vi "ExecutePlay.vi"(0 "object in":refnum<class "StandardAttackPlay.lvclass">, 2 "Robots in":refnum<class "Robot.lvclass">[](array[class]), 3 "GameRef":refnum<data-value>, 5 "error in (no error)":errorcluster) -> (14 "object out":refnum<class "StandardAttackPlay.lvclass">, 16 "Robots out":refnum<class "Robot.lvclass">[](array[class]), 19 "error out":errorcluster)   [LabVIEW 2023, in "StandardAttackPlay.lvclass"]
uses:
  StandardAttackPlay.lvclass
  C:/Users/ebert/Documents/codes/SSL/repo/SSL_AI/NewSTP/NewPlays/Play_v2_class/Play_v2.lvclass
  Robot_class/Robot.lvclass
  Game_class/Game.lvclass
  Play_v2_class/Play_v2.lvclass
  NewRoles/Role_v2_class/Role_v2.lvclass
  Zone_class/Zone.lvclass
  StandardAttackPlay.lvclass/StandardAttackPlay.ctl
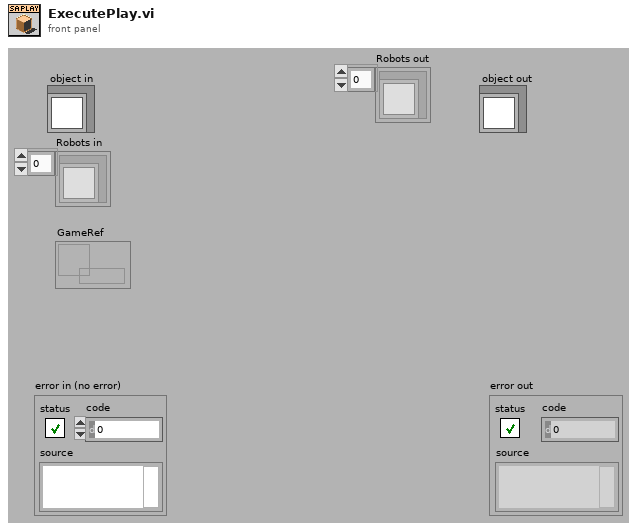
[diagram p1: front panel]
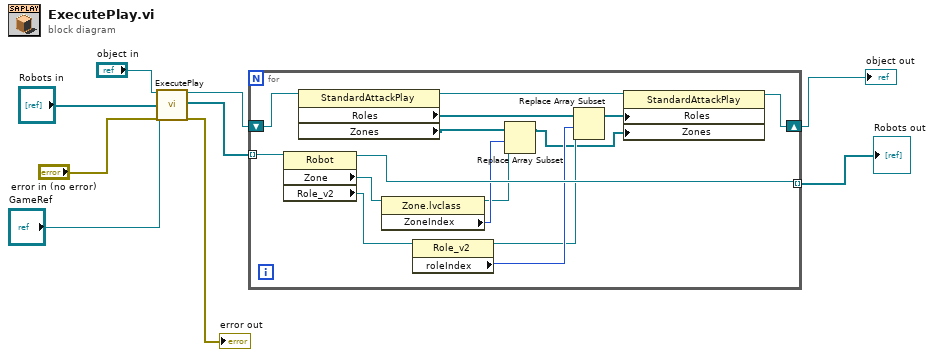
[diagram p0: block diagram]
diagram:
  n1 = call-parent "ExecutePlay.vi"("object in"="object in", "Robots in"="Robots in", "GameRef"="GameRef", "error in (no error)"="error in (no error)") -> ("object out"=w4:refnum<class "StandardAttackPlay.lvclass">, "Robots out"=w5:refnum<class "Robot.lvclass">[], "error out"=→"error out":errorcluster)  [unwired: 13 in]
  n2 = for {
    tunnel: w5 -> [w24] mode=indexing
    tunnel: [w23] -> w3 mode=indexing
    shift-right: [w10] -> w1
    shift-left: w4 -> [w20]
    n3 = property class="Robot"(reference=w24) -> (reference out=w23:refnum<class "Robot.lvclass">, "Zone"=w21:refnum<class "Zone.lvclass">, "Role_v2"=w19:refnum<class "Role_v2.lvclass">)  [unwired: 1 in, 1 out]
    n4 = property class="StandardAttackPlay"(reference=w20) -> (reference out=w11:refnum<class "StandardAttackPlay.lvclass">, "Roles"=w14:refnum<class "Role_v2.lvclass">[], "Zones"=w16:refnum<class "Zone.lvclass">[])  [unwired: 1 in, 1 out]
    n5 = property class="Zone.lvclass"(reference=w21) -> (reference out=w15:refnum<class "Zone.lvclass">, "ZoneIndex"=w22:i32)  [unwired: 1 in, 1 out]
    n6 = property class="Role_v2"(reference=w19) -> (reference out=w17:refnum<class "Role_v2.lvclass">, "roleIndex"=w18:u8)  [unwired: 1 in, 1 out]
    n7 = Replace Array Subset(array=w16, new element=w15, index=w22) -> (w12:refnum<class "Zone.lvclass">[])
    n8 = Replace Array Subset(array=w14, new element=w17, index=w18) -> (w13:refnum<class "Role_v2.lvclass">[])
    n9 = property class="StandardAttackPlay"(reference=w11, "Roles"=w13, "Zones"=w12) -> (reference out=w10:refnum<class "StandardAttackPlay.lvclass">)  [unwired: 1 in, 1 out]
  }
  "object out" <- w1
  "Robots out" <- w3
